vi "ROI_Set_Lock.vi"(0 "error out 2":errorcluster) -> (1 "error out":errorcluster, 2 "Get":bool)   [LabVIEW 2011]
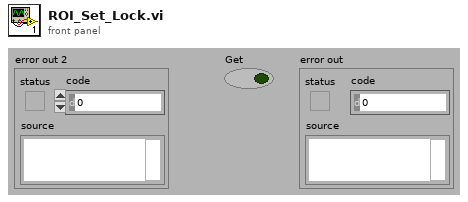
[diagram p1: front panel]
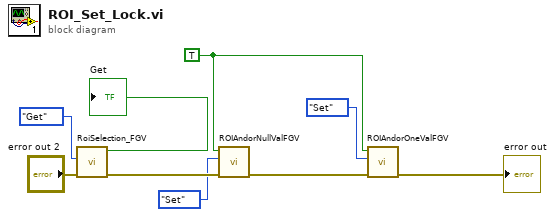
[diagram p0: block diagram]
diagram:
  w1 = TRUE ("set")
  n1 = call "RoiSelection_FGV.vi"("error in"="error out 2", "Set_Get"=enum16{"Set", "Get"}."Get") -> ("error out"=w8:errorcluster, "Get"=→"Get":bool)  [unwired: 8 in]
  n2 = call "ROIAndorNullValFGV.vi"("error in"=w8, "Set_Get"=enum16{"Set", "Get"}."Set", "set"=w1) -> ("error out"=w7:errorcluster)  [unwired: 7 in, 1 out]
  n3 = call "ROIAndorOneValFGV.vi"("error in"=w7, "Set_Get"=enum16{"Set", "Get"}."Set", "set"=w1) -> ("error out"=→"error out":errorcluster)  [unwired: 7 in, 1 out]
